vi "Motor Drive.vi"(8 "Drive Around Mode?":bool=TRUE, 10 "Motor Input":cluster{"Left Drive":dbl, "Right Drive":dbl}, 11 "Enum":enum16{"Init", "Run", "SetBrakeCoast", "End"}(ring)) -> ()   [LabVIEW 2011]
uses:
  <vilib>/Rock Robotics/WPI/CAN/Jaguar/SubVIs/WPI_CANJaguar_BrakeCoastMode.ctl
  <vilib>/Rock Robotics/WPI/CAN/Jaguar/SubVIs/WPI_CANJaguar_ControlMode.ctl
  <vilib>/Rock Robotics/WPI/MotorControl/WPI_MotorControlOpenCANJaguar.vi
  Team Code/Robot Global Data.vi
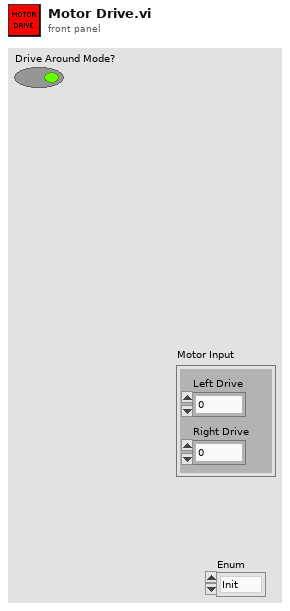
[diagram p1: front panel]
types:
  T1 = typedef "WPI_CANJaguar_BrakeCoastMode.ctl" = enum8{"Jumper", "Brake", "Coast"}
  T2 = typedef "WPI_CANJaguar_ControlMode.ctl" = enum8{"Percent VBus", "Current", "Speed", "Position", "Voltage"}
  T3 = typedef "WPI_MotorControlDeviceRef.ctl" = cluster{"DeviceStatus":errorcluster, "Type":enum16{"PWM", "CAN"}, "PWM":cluster{"Digital Module":T4, "PWM Channel":T5, "DeadBand":T6}, "CAN":cluster{"Device Number":u8, "Control Mode":T2, "Semaphore":T7, "Max Vout":dbl}, "Invert":bool, "TransformRef":T8, "InvTransformRef":T8}
  T4 = typedef "FPGA_TypedefDigitalModule.ctl" = enum16{"Digital Module 1", "Digital Module 2"}
  T5 = typedef "FPGA_DIOPWMChannel.ctl" = enum8{"PWM 1", "PWM 2", "PWM 3", "PWM 4", "PWM 5", "PWM 6", "PWM 7", "PWM 8", "PWM 9", "PWM 10", "Invalid"}
  T6 = typedef "WPI_PWMDeadband.ctl" = cluster{"Name":string, "maxPositivePwm":i32, "minPositivePwm":i32, "centerPwm":i32, "maxNegativePwm":i32, "minNegativePwm":i32, "angularRange":u16}
  T7 = typedef "Semaphore RefNum" = refnum<k1>
  T8 = typedef "WPI_PWMTransform_ConPane.ctl" = refnum<vi>
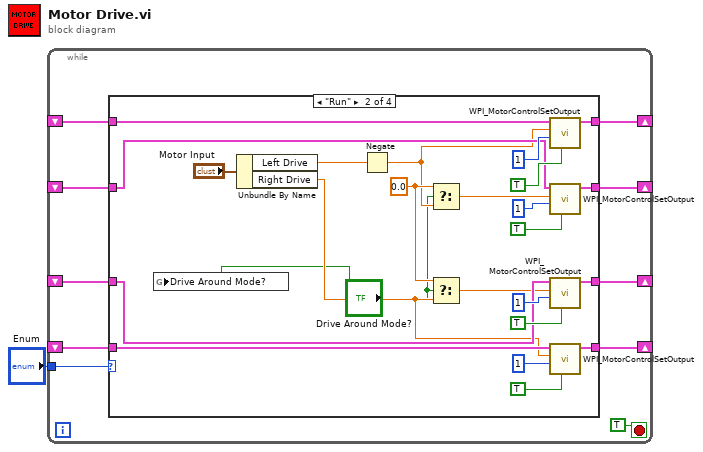
[diagram p0: block diagram]
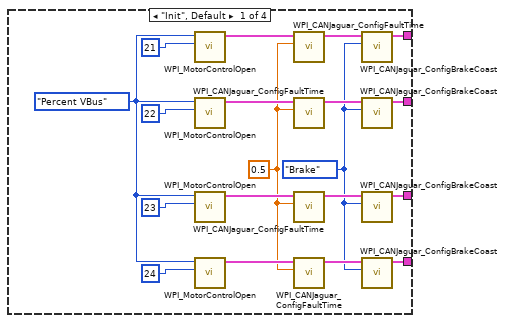
[diagram p2: hidden frame]
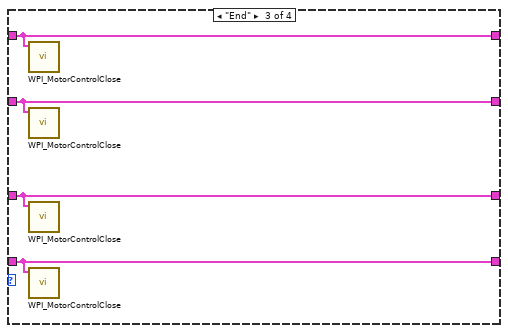
[diagram p3: hidden frame]
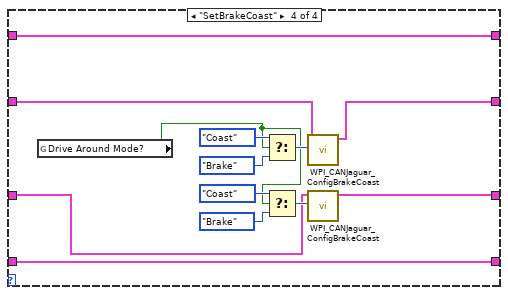
[diagram p4: hidden frame]
diagram:
  n1 = while {
    tunnel: "Enum" -> [w11]
    shift-right: [w10] -> _
    shift-left: _ -> [w8]
    shift-right: [w9] -> _
    shift-left: _ -> [w7]
    shift-right: [w4] -> _
    shift-left: _ -> [w3]
    shift-right: [w5] -> _
    shift-left: _ -> [w2]
    stop <- TRUE stop-if-true
    n2 = case shown="\"Run\"" w11 {
      tunnel: [w14 w44 w58 w65] -> w10
      tunnel: [w15 w43 w57 w61] -> w9
      tunnel: w8 -> [_ w40 w58 w65]
      tunnel: w7 -> [_ w38 w57 w62]
      tunnel: [w17 w42 w56 w60] -> w4
      tunnel: [w18 w41 w55 w64] -> w5
      tunnel: w3 -> [_ w37 w56 w63]
      tunnel: w2 -> [_ w39 w55 w64]
      frame "Init", Default {
        w12 = 0.5 ("Fault Time (s)")
        w13 = WPI_CANJaguar_BrakeCoastMode."Brake" ("Brake / Coast Mode")
        w26 = WPI_CANJaguar_ControlMode."Percent VBus" ("Control Mode")
        n3 = call-poly <vilib>:"WPI_MotorControlOpen.vi"("Device Number"=u8 21, "Control Mode"=w26) -> ("MotorControlDeviceRef"=w21:T3)  [unwired: 8 in, 1 out]
        n4 = call-poly <vilib>:"WPI_MotorControlOpen.vi"("Device Number"=u8 22, "Control Mode"=w26) -> ("MotorControlDeviceRef"=w16:T3)  [unwired: 8 in, 1 out]
        n5 = call-poly <vilib>:"WPI_MotorControlOpen.vi"("Device Number"=u8 23, "Control Mode"=w26) -> ("MotorControlDeviceRef"=w20:T3)  [unwired: 8 in, 1 out]
        n6 = call-poly <vilib>:"WPI_MotorControlOpen.vi"("Device Number"=u8 24, "Control Mode"=w26) -> ("MotorControlDeviceRef"=w19:T3)  [unwired: 8 in, 1 out]
        n7 = call <vilib>:"WPI_CANJaguar_ConfigFaultTime.vi"("Fault Time (s)"=w12, "CAN Jaguar Ref"=w21) -> ("CAN Jaguar Ref Out"=w25:T3)  [unwired: 8 in, 1 out]
        n8 = call <vilib>:"WPI_CANJaguar_ConfigFaultTime.vi"("Fault Time (s)"=w12, "CAN Jaguar Ref"=w16) -> ("CAN Jaguar Ref Out"=w24:T3)  [unwired: 8 in, 1 out]
        n9 = call <vilib>:"WPI_CANJaguar_ConfigFaultTime.vi"("Fault Time (s)"=w12, "CAN Jaguar Ref"=w20) -> ("CAN Jaguar Ref Out"=w23:T3)  [unwired: 8 in, 1 out]
        n10 = call <vilib>:"WPI_CANJaguar_ConfigFaultTime.vi"("Fault Time (s)"=w12, "CAN Jaguar Ref"=w19) -> ("CAN Jaguar Ref Out"=w22:T3)  [unwired: 8 in, 1 out]
        n11 = call <vilib>:"WPI_CANJaguar_ConfigBrakeCoast.vi"("Brake / Coast Mode"=w13, "CAN Jaguar Ref"=w25) -> ("CAN Jaguar Ref Out"=w14:T3)  [unwired: 8 in, 1 out]
        n12 = call <vilib>:"WPI_CANJaguar_ConfigBrakeCoast.vi"("Brake / Coast Mode"=w13, "CAN Jaguar Ref"=w24) -> ("CAN Jaguar Ref Out"=w15:T3)  [unwired: 8 in, 1 out]
        n13 = call <vilib>:"WPI_CANJaguar_ConfigBrakeCoast.vi"("Brake / Coast Mode"=w13, "CAN Jaguar Ref"=w23) -> ("CAN Jaguar Ref Out"=w17:T3)  [unwired: 8 in, 1 out]
        n14 = call <vilib>:"WPI_CANJaguar_ConfigBrakeCoast.vi"("Brake / Coast Mode"=w13, "CAN Jaguar Ref"=w22) -> ("CAN Jaguar Ref Out"=w18:T3)  [unwired: 8 in, 1 out]
      }
      frame "Run" {
        w36 = 0.0 ("t")
        n15 = global write "Robot Global Data.vi" "Drive Around Mode?"("Drive Around Mode?") -> ()
        n16 = Unbundle By Name("Motor Input") -> ("Left Drive"=w45:dbl, "Right Drive"=w34:dbl)
        n17 = Negate(x=w45) -> (-x=w35:dbl)
        n18 = Select(t=w36, s="Drive Around Mode?", f=w35) -> (s? t:f=w32:dbl)
        n19 = Select(t=w36, s="Drive Around Mode?", f=w34) -> (s? t:f=w33:dbl)
        n20 = call <vilib>:"WPI_MotorControlSetOutput.vi"("Isochronous"=TRUE, "Sync Group"=u8 1, "Output"=w35, "MotorControlDevRef"=w40) -> ("MotorControlDevRef"=w44:T3)  [unwired: 6 in, 1 out]
        n21 = call <vilib>:"WPI_MotorControlSetOutput.vi"("Isochronous"=TRUE, "Sync Group"=u8 1, "Output"=w32, "MotorControlDevRef"=w38) -> ("MotorControlDevRef"=w43:T3)  [unwired: 6 in, 1 out]
        n22 = call <vilib>:"WPI_MotorControlSetOutput.vi"("Isochronous"=TRUE, "Sync Group"=u8 1, "Output"=w33, "MotorControlDevRef"=w37) -> ("MotorControlDevRef"=w42:T3)  [unwired: 6 in, 1 out]
        n23 = call <vilib>:"WPI_MotorControlSetOutput.vi"("Isochronous"=TRUE, "Sync Group"=u8 1, "Output"=w34, "MotorControlDevRef"=w39) -> ("MotorControlDevRef"=w41:T3)  [unwired: 6 in, 1 out]
      }
      frame "End" {
        n24 = call <vilib>:"WPI_MotorControlClose.vi"("MotorControlDevRef"=w58) -> ()  [unwired: 10 in, 1 out]
        n25 = call <vilib>:"WPI_MotorControlClose.vi"("MotorControlDevRef"=w57) -> ()  [unwired: 10 in, 1 out]
        n26 = call <vilib>:"WPI_MotorControlClose.vi"("MotorControlDevRef"=w56) -> ()  [unwired: 10 in, 1 out]
        n27 = call <vilib>:"WPI_MotorControlClose.vi"("MotorControlDevRef"=w55) -> ()  [unwired: 10 in, 1 out]
      }
      frame "SetBrakeCoast" {
        n28 = global read "Robot Global Data.vi" "Drive Around Mode?"() -> (w59:bool)
        n29 = Select(t=WPI_CANJaguar_BrakeCoastMode."Coast" ("Brake / Coast Mode 2"), s=w59, f=WPI_CANJaguar_BrakeCoastMode."Brake" ("Brake / Coast Mode 2")) -> (s? t:f=w71:T1)
        n30 = Select(t=WPI_CANJaguar_BrakeCoastMode."Coast" ("Brake / Coast Mode 2"), s=w59, f=WPI_CANJaguar_BrakeCoastMode."Brake" ("Brake / Coast Mode 2")) -> (s? t:f=w68:T1)
        n31 = call <vilib>:"WPI_CANJaguar_ConfigBrakeCoast.vi"("Brake / Coast Mode"=w71, "CAN Jaguar Ref"=w62) -> ("CAN Jaguar Ref Out"=w61:T3)  [unwired: 8 in, 1 out]
        n32 = call <vilib>:"WPI_CANJaguar_ConfigBrakeCoast.vi"("Brake / Coast Mode"=w68, "CAN Jaguar Ref"=w63) -> ("CAN Jaguar Ref Out"=w60:T3)  [unwired: 8 in, 1 out]
      }
    }
  }
